vi "Write_lastpoint.vi"(2 "error in (no error)":errorcluster caption="错误输入（无错误）", 3 "小平台X轴正限位mm":dbl=4000.0, 4 "工位写入":cluster{"字符串":string, "数值":i32}[](array[cluster]), 5 "本次位置数据":i32[](array[numeric]), 6 "坐标位置":dbl[][](array[numeric]), 7 "Jog.csv":path caption="文件路径 （空时为对话框）") -> (0 "error out":errorcluster caption="错误输出")   [LabVIEW 2018]
uses:
  <vilib>/Utility/file.llb/Write Delimited Spreadsheet (DBL).vi
  <vilib>/Utility/file.llb/Write Delimited Spreadsheet (string).vi
panel:
  out "添加的数组":dbl[][](array[numeric])
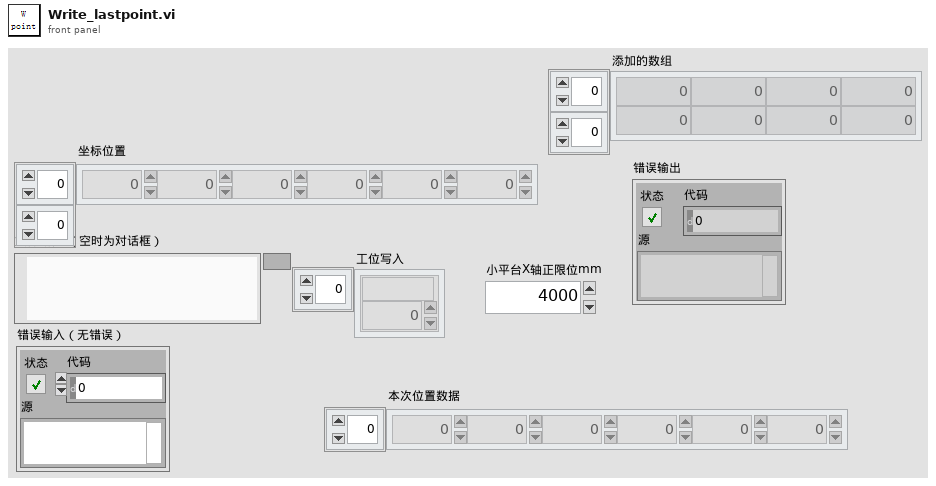
[diagram p1: front panel]
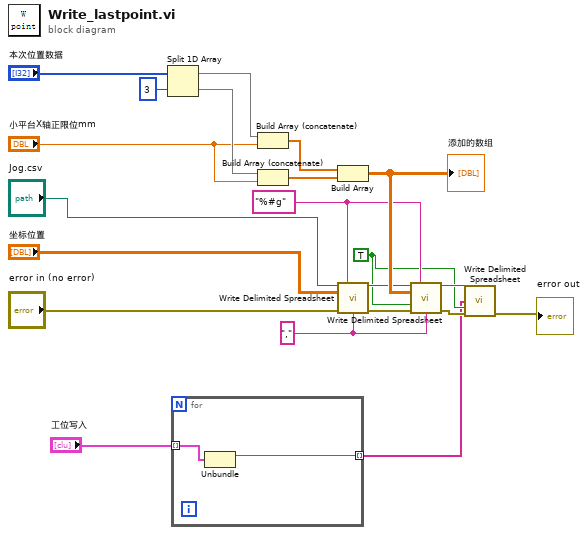
[diagram p0: block diagram]
diagram:
  w14 = "," ("delimiter (\\t)")
  w16 = "%#g" ("format (%.3f)")
  w4 = TRUE ("append to file? (new file:F)")
  n1 = Split 1D Array(array="本次位置数据", index=3 ("索引")) -> (first subarray=w12:i32[], second subarray=w11:i32[])
  n2 = for {
    tunnel: "工位写入" -> [w23] mode=indexing
    tunnel: [w22] -> w1 mode=indexing
    n3 = Unbundle(w23) -> ("字符串"=w22:string)  [unwired: 1 out]
  }
  n4 = Build Array (concatenate)(w12, "小平台X轴正限位mm") -> (w9:dbl[])
  n5 = Build Array (concatenate)(w11, "小平台X轴正限位mm") -> (w8:dbl[])
  n6 = Build Array(w9, w8) -> (w19:dbl[][])
  "添加的数组" <- w19
  n7 = call-poly <vilib>:"Write Delimited Spreadsheet.vi"("file path (dialog if empty)"="Jog.csv", "format (%.3f)"=w16, "2D data"="坐标位置", "error in (no error)"="error in (no error)", "delimiter (\\t)"=w14) -> ("new file path (Not A Path if cancelled)"=w17:path, "error out"=w13:errorcluster)  [unwired: 9 in]
  n8 = call-poly <vilib>:"Write Delimited Spreadsheet.vi"("file path (dialog if empty)"=w17, "format (%.3f)"=w16, "2D data"=w19, "append to file? (new file:F)"=w4, "error in (no error)"=w13, "delimiter (\\t)"=w14) -> ("new file path (Not A Path if cancelled)"=w6:path, "error out"=w5:errorcluster)  [unwired: 8 in]
  n9 = call-poly <vilib>:"Write Delimited Spreadsheet.vi"("file path (dialog if empty)"=w6, "1D data"=w1, "append to file? (new file:F)"=w4, "error in (no error)"=w5) -> ("error out"=→"error out":errorcluster)  [unwired: 10 in, 1 out]
